vi "PR4000 set wait after set.vi"(8 "error in (no error)":errorcluster, 10 "Channel parsed command info":T1, 11 "MKS4000b in":refnum<class "MKS4000b.lvclass">) -> (0 "error out":errorcluster, 2 "new commands":string, 3 "MKS4000b out":refnum<class "MKS4000b.lvclass">)   [LabVIEW 2020, in "MKS4000b.lvclass"]
uses:
  MKS4000b.lvclass
  channel parsed cmd cluster.ctl
  MKS4000b.lvclass/MKS4000b.ctl
  CompressAndUpdate(Numeric).vi
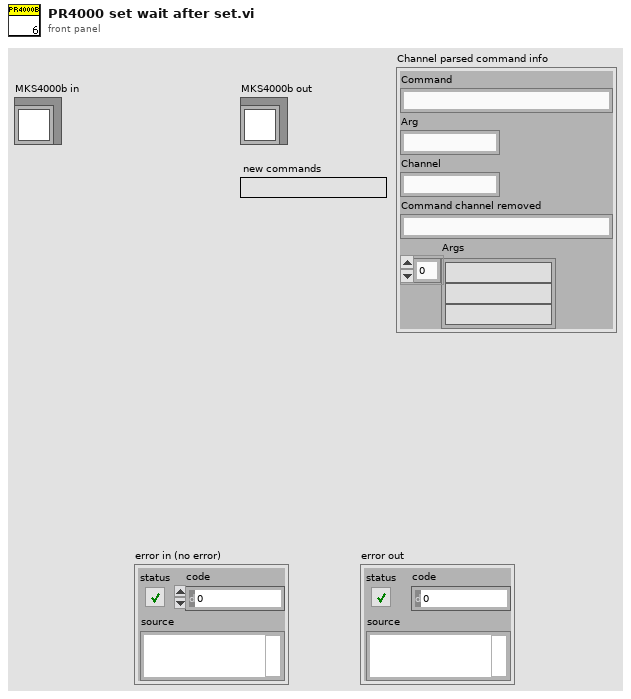
[diagram p1: front panel]
types:
  T1 = typedef "channel parsed cmd cluster.ctl" = cluster{"Command":string, "Arg":string, "Channel":string, "Command channel removed":string, "Args":string[]}
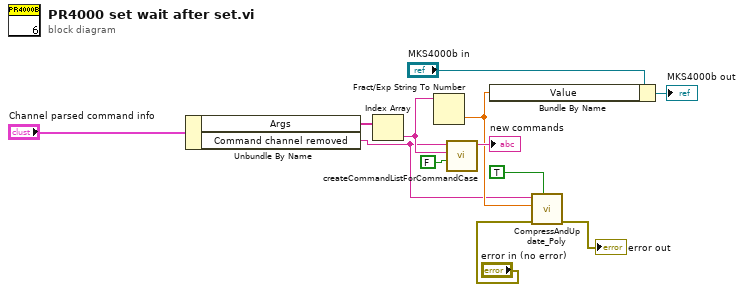
[diagram p0: block diagram]
diagram:
  n1 = Unbundle By Name("Channel parsed command info") -> ("Args"=w4:string[], "Command channel removed"=w3:string)
  n2 = Index Array(array=w4) -> (element=w8:string)  [unwired: 1 in]
  n3 = Fract/Exp String To Number(string=w8) -> (number=w10:dbl)  [unwired: 3 in, 1 out]
  n4 = call "createCommandListForCommandCase.vi"("immediate Check (only once)"=FALSE, "setvalue"=w8, "command"=w3) -> ("new commands"=→"new commands":string)  [unwired: 8 in]
  n5 = Bundle By Name(cluster="MKS4000b in", "Value"=w10) -> (→"MKS4000b out":refnum<class "MKS4000b.lvclass">)
  n6 = call-poly "CompressAndUpdate_Poly.vi"("force CVT update (false)"=TRUE ("force CVT update"), "error in"="error in (no error)", "Numeric"=w10, "command or variable name"=w3) -> ("error out"=→"error out":errorcluster)  [unwired: 7 in]
